vi "T_Sat_Curve_Fit_R134a-for_doubles.vi"(8 "error in (no error)":errorcluster, 11 "Numeric in":dbl) -> (0 "error out":errorcluster, 3 "Numeric out":dbl)   [LabVIEW 2016]
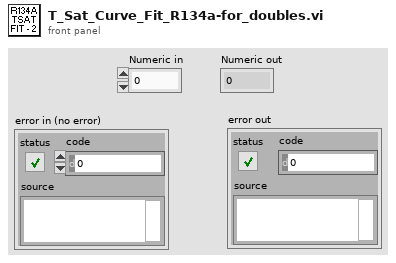
[diagram p1: front panel]
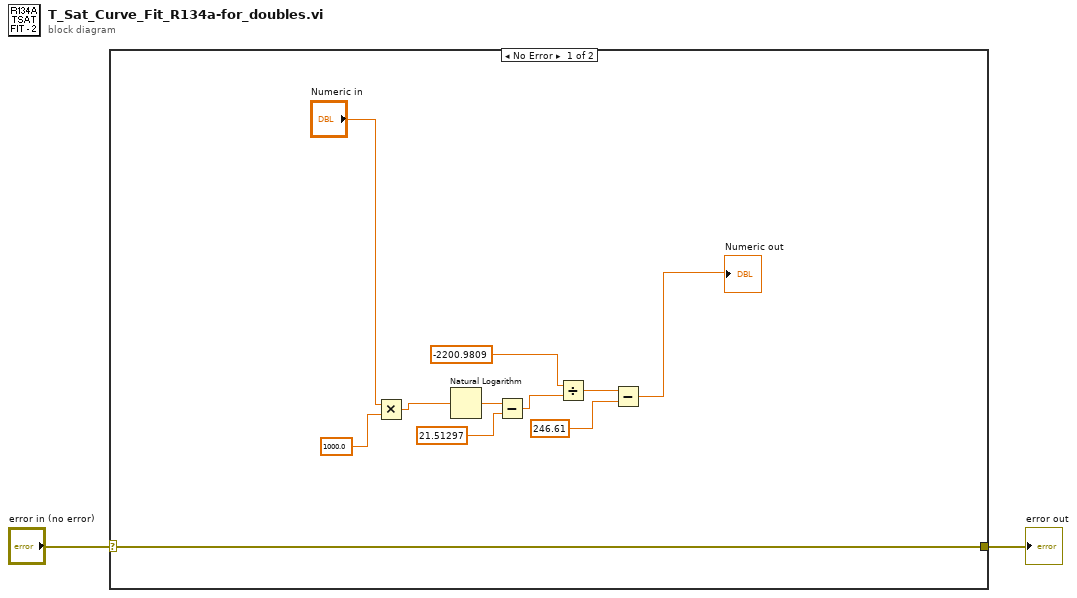
[diagram p0: block diagram]
diagram:
  n1 = case shown="No Error" "error in (no error)" {
    selector: "error in (no error)" -> [w3 w14]
    tunnel: [w3 w14] -> w1
    frame No Error {
      n2 = Multiply(x="Numeric in", y=1000.0) -> (x*y=w5:dbl)
      n3 = Natural Logarithm(1:w5) -> (0:w6:dbl)
      n4 = Subtract(x=w6, y=21.51297) -> (x-y=w9:dbl)
      n5 = Divide(x=-2200.9809, y=w9) -> (x/y=w10:dbl)
      n6 = Subtract(x=w10, y=246.61) -> (x-y=→"Numeric out":dbl)
    }
    frame Error {
    }
  }
  "error out" <- w1
